vi "Close RxTx.vi"(8 "error in (no error)":errorcluster, 11 "Roda_Filtros in":refnum<class "Roda_Filtros.lvclass">) -> (0 "error out":errorcluster, 3 "Roda_Filtros out":refnum<class "Roda_Filtros.lvclass">)   [LabVIEW 2018, in "Roda_Filtros.lvclass"]
uses:
  Roda_Filtros.lvclass
  Roda_Filtros.lvclass/Roda_Filtros.ctl
  RxTx/RxTx.lvclass
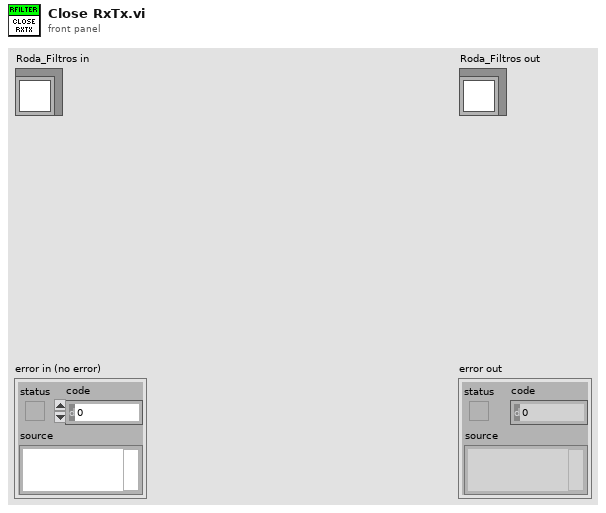
[diagram p1: front panel]
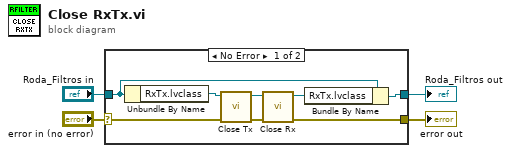
[diagram p0: block diagram]
diagram:
  n1 = case shown="No Error" "error in (no error)" {
    selector: "error in (no error)" -> [w9 w14]
    tunnel: [w10 w14] -> w3
    tunnel: [w6 w13] -> w1
    tunnel: "Roda_Filtros in" -> [w7 w13]
    frame No Error {
      n2 = Unbundle By Name(w7) -> ("RxTx.lvclass"=w8:refnum<class "RxTx.lvclass">)
      n3 = call "Close Tx.vi"("error in (no error)"=w9, "RxTx in"=w8) -> ("error out"=w12:errorcluster, "RxTx out"=w11:refnum<class "RxTx.lvclass">)  [unwired: 8 in]
      n4 = call "Close Rx.vi"("error in (no error)"=w12, "RxTx in"=w11) -> ("error out"=w10:errorcluster, "RxTx out"=w5:refnum<class "RxTx.lvclass">)  [unwired: 8 in]
      n5 = Bundle By Name(cluster=w7, "RxTx.lvclass"=w5) -> (w6:refnum<class "Roda_Filtros.lvclass">)
    }
    frame Error {
    }
  }
  "error out" <- w3
  "Roda_Filtros out" <- w1
